vi "Mixed1.vi"() -> ()   [LabVIEW 2013]
uses:
  <vilib>/sound2/lvsound2.llb/Sampling Mode.ctl
  <vilib>/sound2/lvsound2.llb/Sound Data Format.ctl
  <vilib>/measure/maspectr.llb/Power Spectrum and PSD Export Mode.ctl
  <vilib>/Analysis/4window.llb/windowTd.ctl
  <vilib>/measure/maspectr.llb/FFT Power Spectrum and PSD for N Chan.vi
  <vilib>/measure/maspectr.llb/FFT Spectrum (Mag-Phase) for N Chan.vi
  <vilib>/sound2/lvsound2.llb/Sound Output Set Volume (Single).vi
  <vilib>/sound2/lvsound2.llb/Sound Output Write (DBL Single).vi
  <vilib>/Analysis/NI_AALBase.lvlib
  <vilib>/measure/NI_MAPro.lvlib
  <vilib>/Analysis/NI_AALPro.lvlib
panel:
  in  "Volume":dbl(knob)=50.0 scale=0.0..100.0
  in  "Device ID":u32
  out "Signal Generated":T1(graph)={0.0, 0.01, "arbitrary wave"=[]}
  in  "Frequency Unit":u16(ring) items=["Hz", "cycles"]
  in  "Reset phase":bool
  in  "Sampling rate (Hz)":dbl(knob)=100.0 step=1.0 scale=0.0..100.0
  out "Waveform Pattern":dbl[](graph)
  in  "interpolation":i32(ring)=1 items=["none", "linear"]
  in  "Wave Table":dbl[](array[knob])=[0.0, 1.0, 4.0, 0.2, -0.9] scale=0.0..10.0
  in  "Sine":bool caption="Enable"
  in  "Frequency":dbl(knob) scale=0.0..1000.0
  in  "Arbitary":bool
  in  "Blank Button 7":bool
  in  "Clear":bool
  in  "Blank Button 5":bool
  in  "Sawtooth":bool
  in  "Triangle":bool
  in  "Square":bool
  in  "Delay":dbl(knob) scale=0.0..3000.0
  in  "?":dbl(knob) scale=0.0..10.0
  out "Waveform Graph 5":dynamicdata(graph)
  out "Waveform Graph 3":cluster{"f0":dbl, "df":dbl, "magnitude":dbl[]}[](graph)
  out "Waveform Graph":cluster{"f0":dbl, "df":dbl, "magnitude":dbl[]}[](graph)
  in  "Amplitude":dbl(knob) scale=0.0..10.0
  in  "Phase":dbl(knob) scale=0.0..10.0
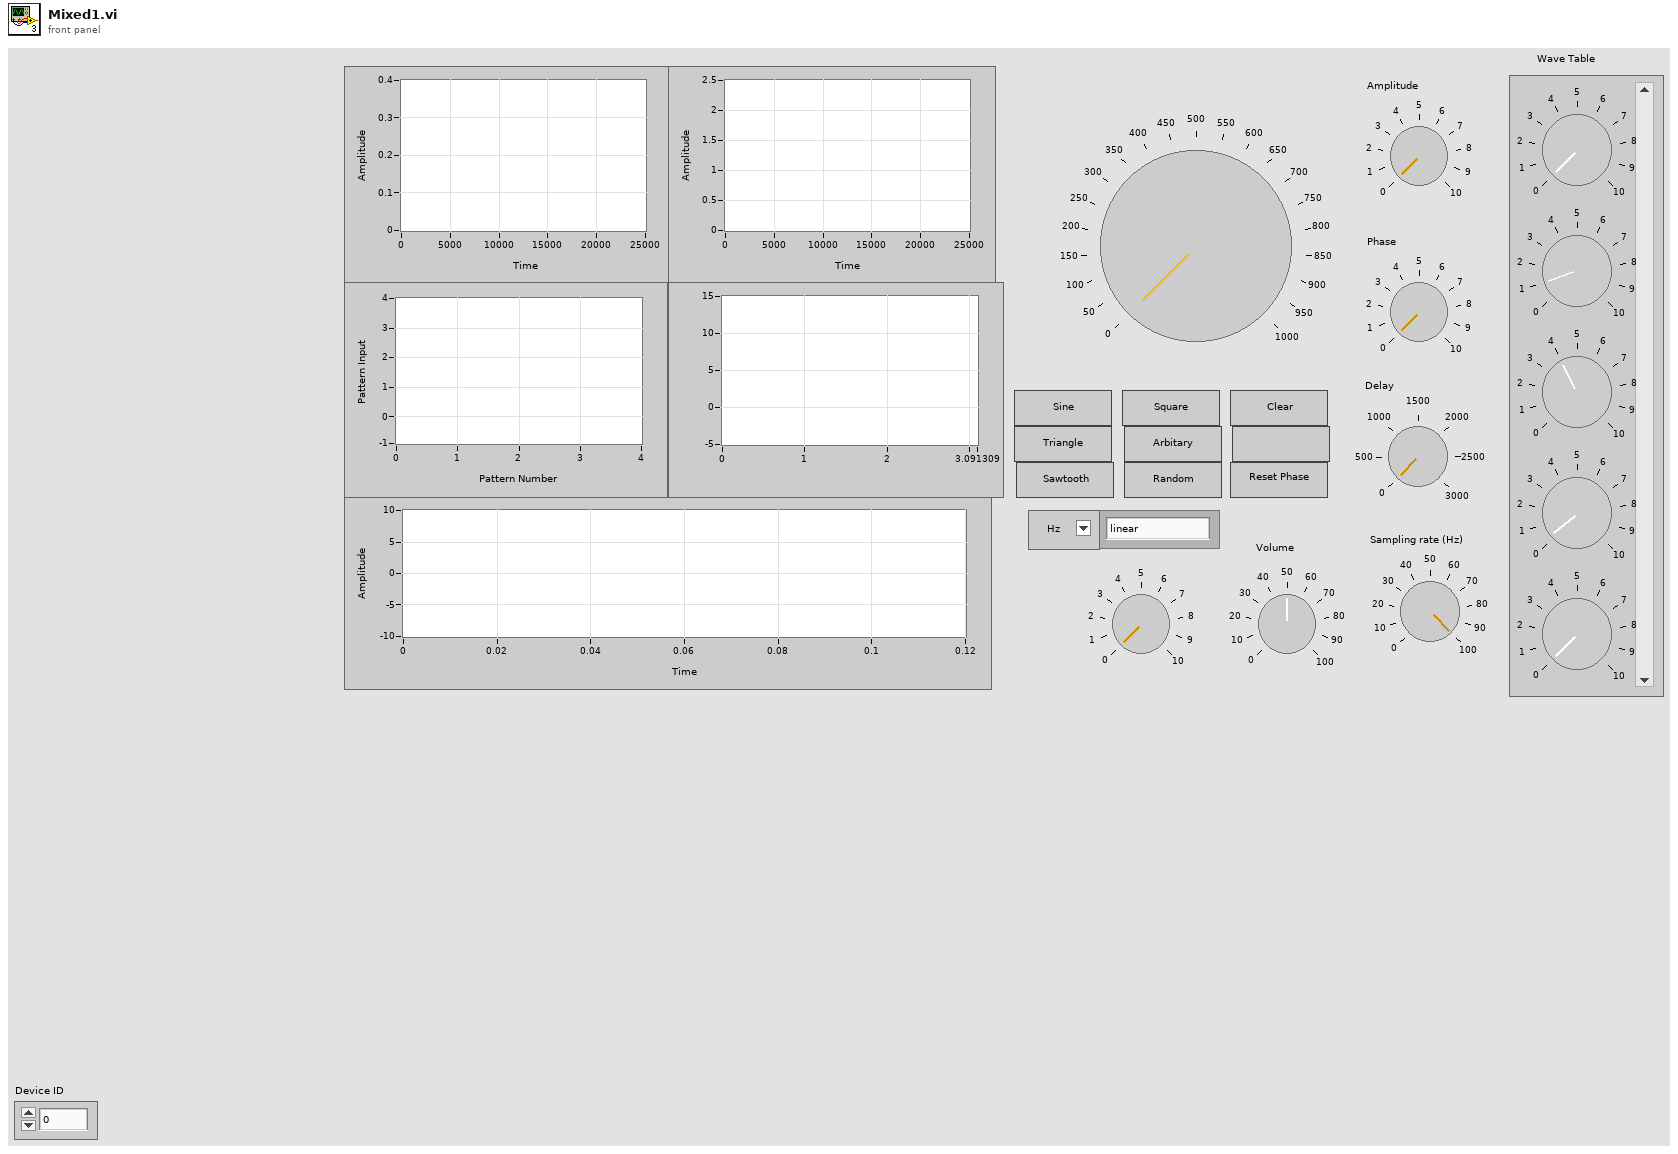
[diagram p1: front panel]
types:
  T1 = cluster{dbl[unit], dbl[unit], "arbitrary wave":dbl[]}
  T2 = typedef "Sound Data Format.ctl" = cluster{"sample rate (S/s)":dbl, "number of channels":i32, "bits per sample":i32}
  T3 = typedef "Sampling Mode.ctl" = i32
  T4 = typedef "Sound Output Task ID.ctl" = u32
  T5 = cluster{"dB On (F)":bool, "unwrap phase (F)":bool, "convert to degree (F)":bool}
  T6 = cluster{"averaging mode":enum16{"No averaging", "Vector averaging", "RMS averaging", "Peak hold"}, "weighting mode":enum16{"Linear", "Exponential"}, "number of averages":u32}
  T7 = typedef "NI_AALPro.lvlib/windowTd.ctl" = u32
  T8 = typedef "NI_MAPro.lvlib/Power Spectrum and PSD Export Mode.ctl" = u16
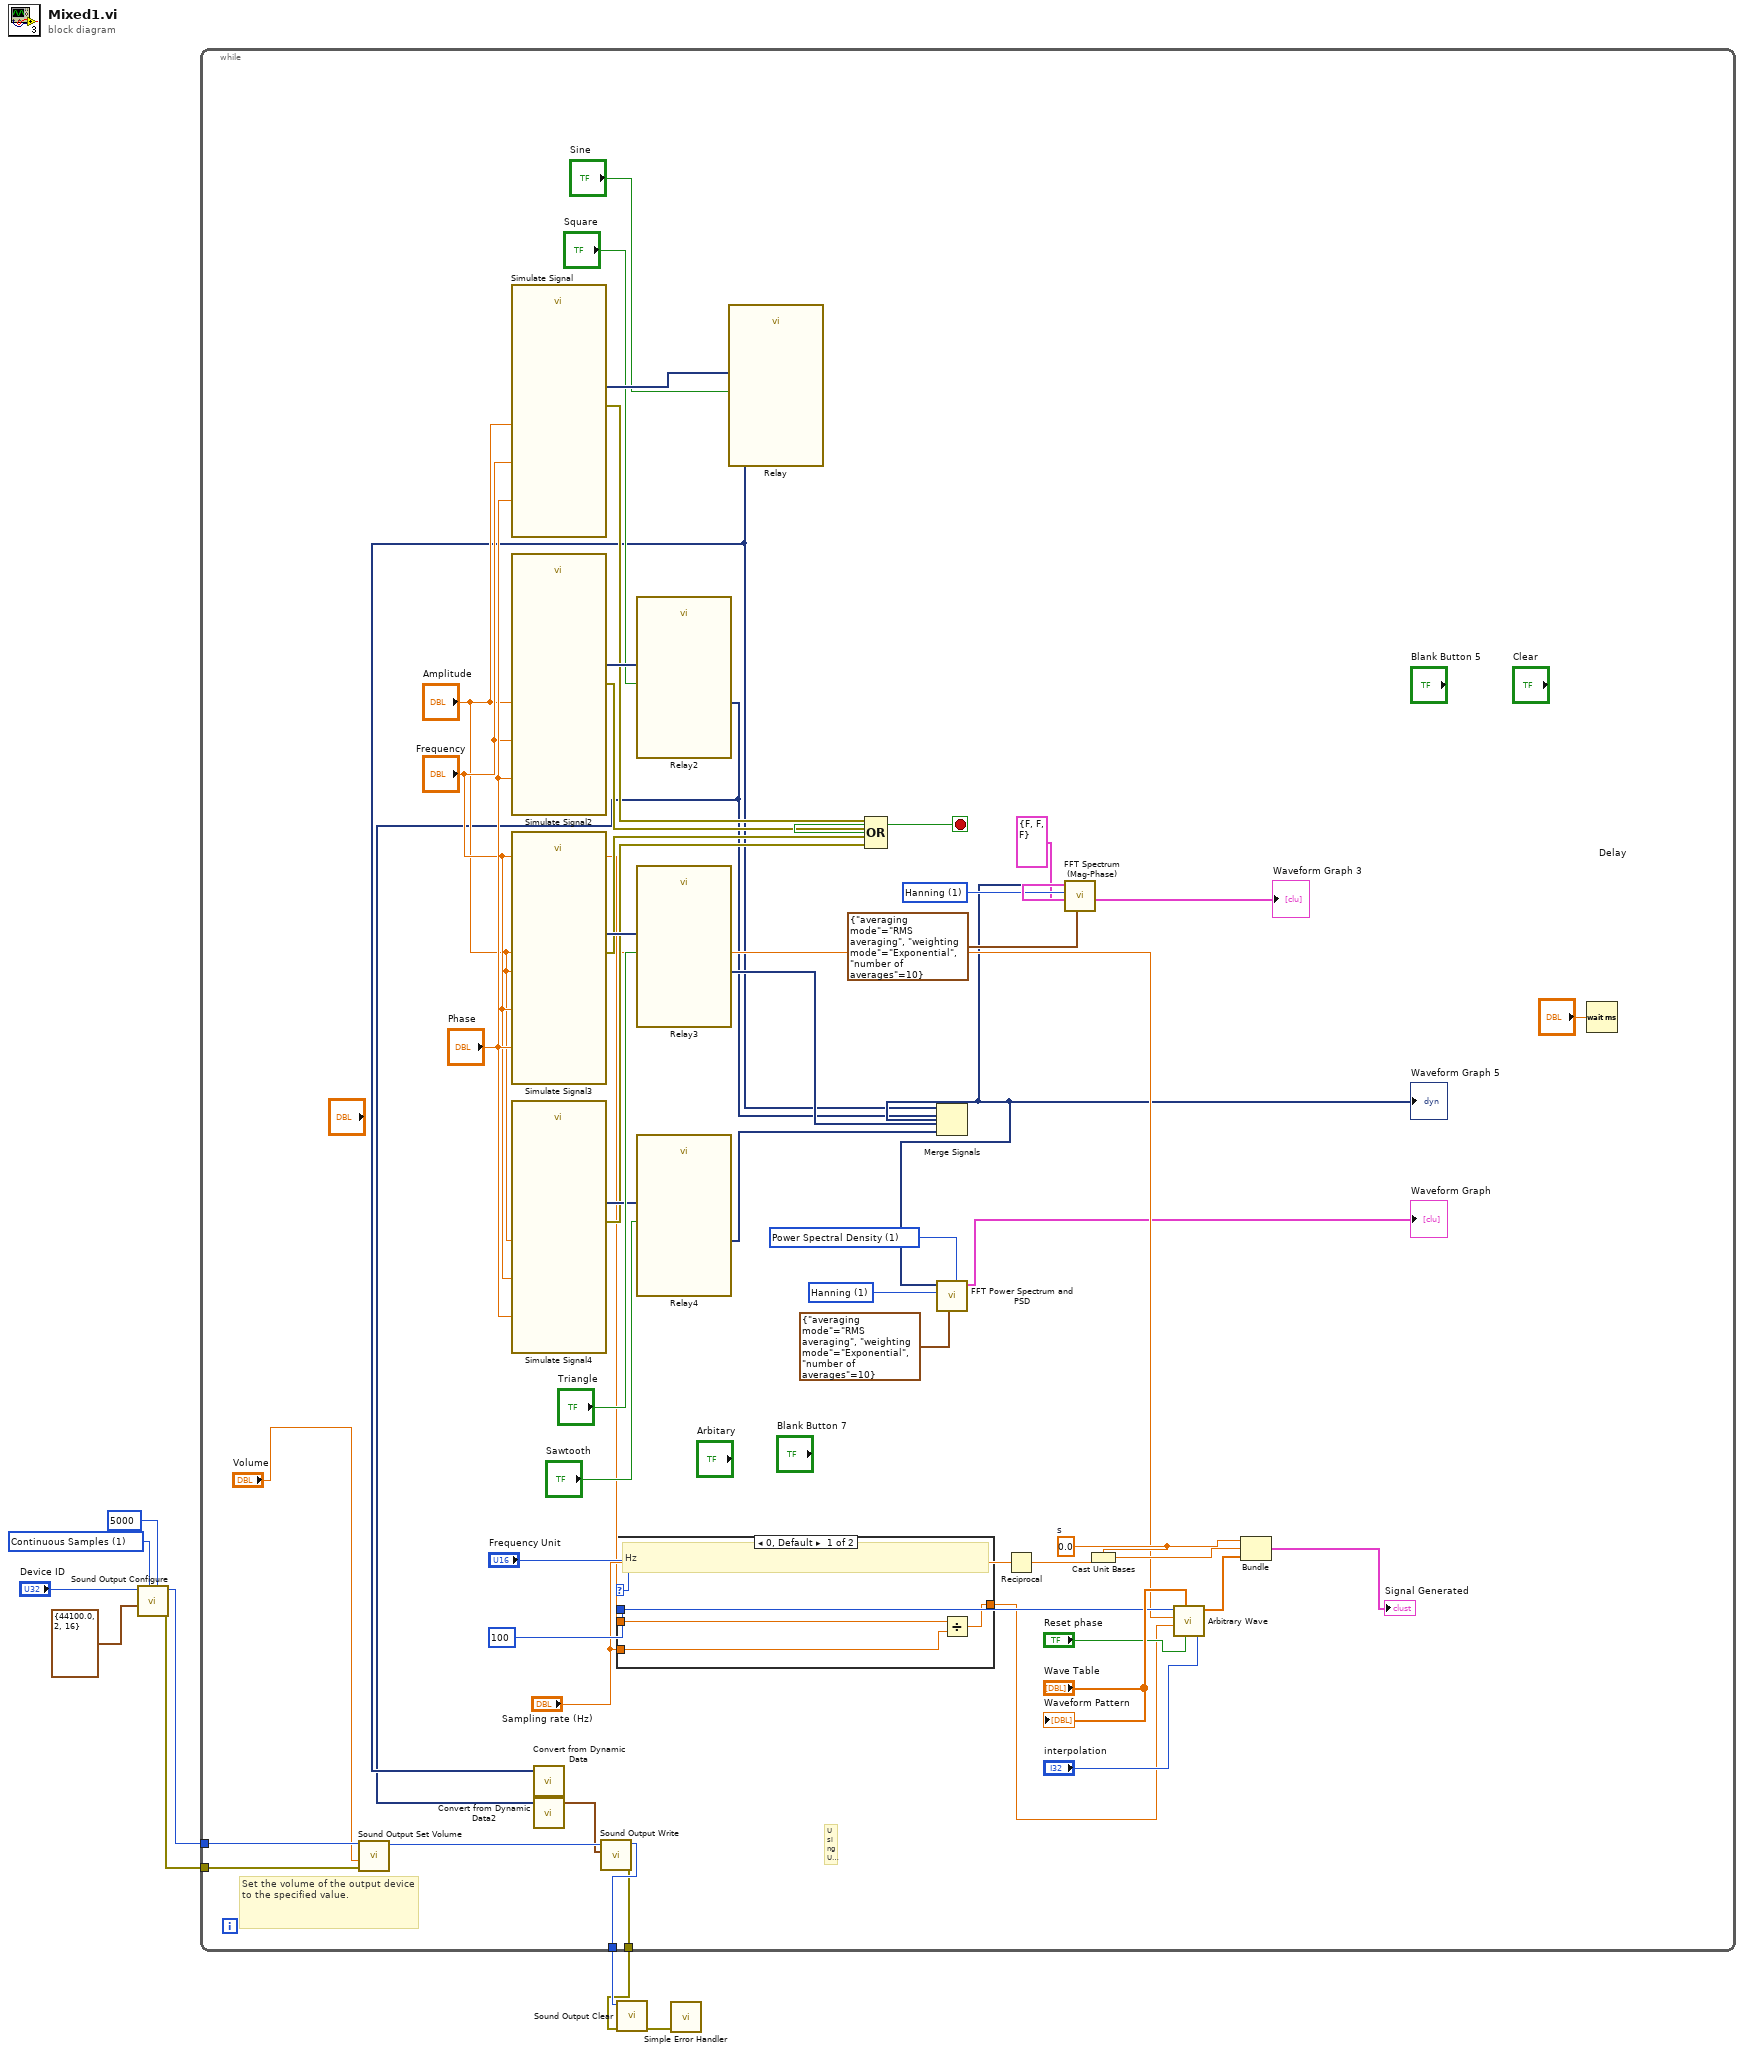
[diagram p0: block diagram]
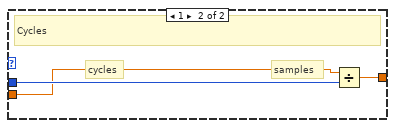
[diagram p2: hidden frame]
diagram:
  w8 = T3 1 items=["Finite Samples", "Continuous Samples"] ("sample mode")
  n1 = call <vilib>:"Sound Output Configure.vi"("number of samples/ch"=5000 ("Number of Samples/ch"), "sample mode"=w8, "sound format"=T2 {"sample rate (S/s)"=44100.0, "number of channels"=2, "bits per sample"=16} ("Sound Format"), "device ID"="Device ID") -> ("error out"=w4:errorcluster, "task ID"=w5:T4)  [unwired: 6 in]
  n2 = while {
    tunnel: w5 -> [w18]
    tunnel: w4 -> [w17]
    tunnel: [w16] -> w2
    tunnel: [w15] -> w1
    stop <- w46 stop-if-true
    w23 = T7 1 items=["Rectangle"=0, "Hanning"=1, "Hamming"=2, "Blackman-Harris"=3, "Exact Blackman"=4, "Blackman"=5, "Flat Top"=6, "4 Term B-Harris "=7, "7 Term B-Harris"=8, "Low Sidelobe"=9, "Blackman Nuttall"=11, "Triangle"=30, "Bartlett-Hanning"=31, "Bohman"=32, "Parzen"=33, "Welch"=34, "Kaiser"=60, "Dolph-Chebyshev"=61, "Gaussian"=62] ("window")
    w25 = T7 1 items=["Rectangle"=0, "Hanning"=1, "Hamming"=2, "Blackman-Harris"=3, "Exact Blackman"=4, "Blackman"=5, "Flat Top"=6, "4 Term B-Harris "=7, "7 Term B-Harris"=8, "Low Sidelobe"=9, "Blackman Nuttall"=11, "Triangle"=30, "Bartlett-Hanning"=31, "Bohman"=32, "Parzen"=33, "Welch"=34, "Kaiser"=60, "Dolph-Chebyshev"=61, "Gaussian"=62] ("window")
    w26 = T8 1 items=["Power Spectrum", "Power Spectral Density"] ("export mode")
    w33 = dbl[unit] 0.0  # s
    w40 = 100 ("samples")
    # "Set the volume of the output device to the specified value."
    # "Using Unit in datatype"
    n3 = call-poly <vilib>:"Sound Output Set Volume.vi"("error in (no error)"=w17, "volume"="Volume", "task ID"=w18) -> ("task ID out"=w19:T4)  [unwired: 7 in, 1 out]
    n4 = call "Simulate Signal"("Frequency"="Frequency", "Amplitude"="Amplitude", "Phase"="Phase") -> ("Sine"=w57:dynamicdata, "error out"=w45:errorcluster)  [unwired: 11 in]
    n5 = call "Simulate Signal2"("Frequency"="Frequency", "Amplitude"="Amplitude", "Phase"="Phase") -> ("Square"=w55:dynamicdata, "error out"=w44:errorcluster)  [unwired: 11 in]
    n6 = call "Simulate Signal3"("Frequency"="Frequency", "Amplitude"="Amplitude", "Phase"="Phase") -> ("Triangle"=w53:dynamicdata, "error out"=w43:errorcluster)  [unwired: 11 in]
    n7 = call "Simulate Signal4"("Frequency"="Frequency", "Amplitude"="Amplitude", "Phase"="Phase") -> ("Sawtooth"=w50:dynamicdata, "error out"=w42:errorcluster)  [unwired: 11 in]
    n8 = case shown="0, Default" "Frequency Unit" {
      tunnel: [w61 w63] -> w31
      tunnel: w40 -> [_ w64]
      tunnel: "Frequency" -> [w60 w62]
      tunnel: "Sampling rate (Hz)" -> [w59 _]
      frame 0, Default {
        # "Hz"
        n9 = Divide(x=w60, y=w59) -> (x/y=w61:dbl)
      }
      frame 1 {
        # "samples"
        # "cycles"
        # "Cycles"
        n10 = Divide(x=w62, y=w64) -> (x/y=w63:dbl)
      }
    }
    n11 = call "Relay2"("Enable"="Square", "Signals"=w55) -> ("Result"=w11:dynamicdata)  [unwired: 8 in, 1 out]
    n12 = call "Convert from Dynamic Data2"("Dynamic Data Type"=w11) -> ("Waveform"=w10:waveform(dbl))  [unwired: 3 in]
    n13 = call-poly <vilib>:"Sound Output Write.vi"("data"=w10, "task ID"=w19) -> ("error out"=w15:errorcluster, "task ID out"=w16:T4)  [unwired: 8 in]
    n14 = call "Relay3"("Enable"="Triangle", "Signals"=w53) -> ("Result"=w49:dynamicdata)  [unwired: 8 in, 1 out]
    n15 = call "Relay4"("Enable"="Sawtooth", "Signals"=w50) -> ("Result"=w48:dynamicdata)  [unwired: 8 in, 1 out]
    n16 = call "Relay"("Enable"="Sine", "Signals"=w57) -> ("Result"=w12:dynamicdata)  [unwired: 8 in, 1 out]
    n17 = call "Convert from Dynamic Data"("Dynamic Data Type"=w12) -> ()  [unwired: 3 in, 1 out]
    n18 = Compound Arithmetic op=OR(w45, w44, w43, w42) -> (w46:bool)
    n19 = Merge Signals(w12, w11, w49, w48) -> (w13:dynamicdata)
    "Waveform Graph 5" <- w13
    n20 = call-poly <vilib>:"FFT Power Spectrum and PSD.vi"("export mode"=w26, "averaging parameters"=T6 {"averaging mode"=enum."RMS averaging", "weighting mode"=enum."Exponential", "number of averages"=10}, "window"=w25, "time signals"=w13) -> ("Power Spectrum / PSD"=→"Waveform Graph":cluster{"f0":dbl, "df":dbl, "magnitude":dbl[]}[])  [unwired: 4 in, 3 out]
    n21 = Reciprocal(x="Sampling rate (Hz)") -> (1/x=w36:dbl)
    n22 = call-poly <vilib>:"FFT Spectrum (Mag-Phase).vi"("averaging parameters"=T6 {"averaging mode"=enum."RMS averaging", "weighting mode"=enum."Exponential", "number of averages"=10}, "view"=T5 {"dB On (F)"=FALSE, "unwrap phase (F)"=FALSE, "convert to degree (F)"=FALSE}, "window"=w23, "time signals"=w13) -> ("magnitudes"=→"Waveform Graph 3":cluster{"f0":dbl, "df":dbl, "magnitude":dbl[]}[])  [unwired: 3 in, 4 out]
    n23 = Cast Unit Bases(0:w36, 1:w33) -> (2:w35:dbl[unit])
    n24 = call <vilib>:"Arbitrary Wave.vi"("interpolation"="interpolation", "reset phase"="Reset phase", "Wave Table"="Wave Table", "frequency"=w31, "amplitude"="Amplitude", "samples"=w40) -> ("arbitrary wave"=w37:dbl[])  [unwired: 1 in, 2 out]
    n25 = Bundle(w33, w35, "arbitrary wave"=w37) -> (→"Signal Generated":T1)  [unwired: 1 in]
    n26 = Wait (ms)(milliseconds to wait="Delay") -> ()  [unwired: 1 out]
    "Waveform Pattern" <- "Wave Table"
  }
  n27 = call <vilib>:"Sound Output Clear.vi"("error in (no error)"=w1, "task ID"=w2) -> ("error out"=w3:errorcluster)  [unwired: 9 in]
  n28 = call <vilib>:"Simple Error Handler.vi"("error in (no error)"=w3) -> ()  [unwired: 4 in, 5 out]
